vi "Controle_velocidade_servo_SubVI.vi"(9 "Posição Desejada":dbl, 10 "Posição":dbl, 11 "milliseconds to wait":u32) -> (2 "Duty Cycle":dbl(slide)=1.5 scale=0.025..0.125, 3 "Posição":dbl(knob)=1.5 scale=0.0..200.0)   [LabVIEW 2017]
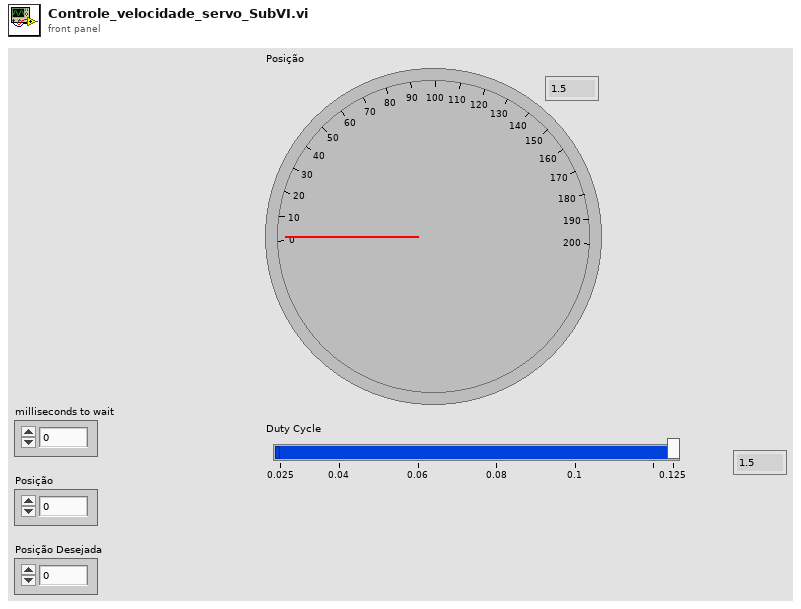
[diagram p1: front panel]
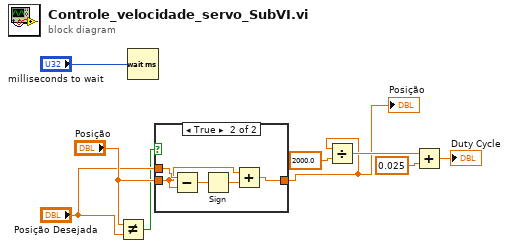
[diagram p0: block diagram]
diagram:
  n1 = Not Equal?(x="Posição", y="Posição Desejada") -> (x != y?=w1:bool)
  n2 = Wait (ms)(milliseconds to wait="milliseconds to wait") -> ()  [unwired: 1 out]
  n3 = case shown="True" w1 {
    tunnel: "Posição Desejada" -> [_ w15]
    tunnel: "Posição" -> [w10 w13]
    tunnel: [w10 w12] -> w2
    frame False {
    }
    frame True {
      n4 = Subtract(x=w15, y=w13) -> (x-y=w14:dbl)
      n5 = Sign(1:w14) -> (0:w11:dbl)
      n6 = Add(x=w13, y=w11) -> (x+y=w12:dbl)
    }
  }
  "Posição" <- w2
  n7 = Divide(x=w2, y=2000.0) -> (x/y=w5:dbl)
  n8 = Add(x=w5, y=0.025) -> (x+y=→"Duty Cycle":dbl)
